vi "To Variant.vi"(8 "error in (no error)":errorcluster, 11 "Abs_Time in":refnum<class "Abs_Time.lvclass">) -> (0 "error out":errorcluster, 2 "Variant":variant, 3 "Abs_Time out":refnum<class "Abs_Time.lvclass">)   [LabVIEW 2021, in "Abs_Time.lvclass"]
uses:
  Abs_Time.lvclass
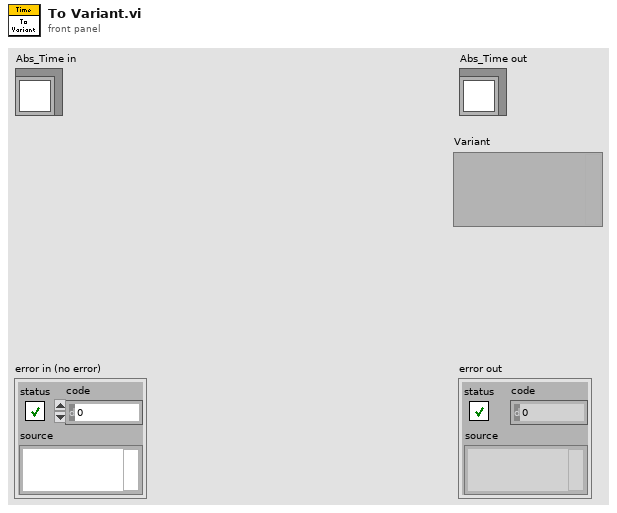
[diagram p1: front panel]
types:
  T1 = typedef "Abs_Time.lvclass/Type.ctl" = timestamp
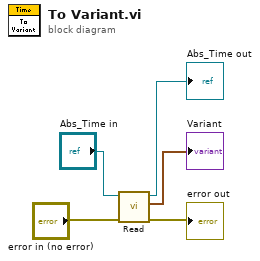
[diagram p0: block diagram]
diagram:
  n1 = call-dynamic "Read.vi"("error in (no error)"="error in (no error)", "Double Float.lvclass_340760 in"="Abs_Time in") -> ("error out"=→"error out":errorcluster, "Value"=→"Variant":T1, "Double Float.lvclass_340760 out"=→"Abs_Time out":refnum<class "Abs_Time.lvclass">)  [unwired: 7 in]
